vi "SFC_Get Model Label Template.vi"(8 "error in (no error)":errorcluster caption="错误输入（无错误）", 10 "Model":string, 11 "Traceability 引用句柄":refnum<k24>) -> (0 "error out":errorcluster caption="错误输出", 2 ".NET:System.Data.DataSet":T1={"CaseSensitive"=FALSE, "Container"=refnum, "DataSetName"="", "DefaultViewManager"=refnum, "DesignMode"=FALSE, "EnforceConstraints"=FALSE, "ExtendedProperties"=refnum, "HasErrors"=FALSE, "IsInitialized"=FALSE, "Locale"=refnum, "Namespace"="", "Prefix"="", "Relations"=refnum, "RemotingFormat"=0, "SchemaSerializationMode"=1, "Site"=refnum, "Tables"=refnum} {"SchemaSerializationMode" items=["IncludeSchema"=1, "ExcludeSchema"=2]; "RemotingFormat" items=["Xml", "Binary"]}, 3 "Traceability 引用句柄输出":refnum<k24>)   [LabVIEW 2014, in "Traceability.lvlib"]
uses:
  D:/webservice/Traceability.dll
  Traceability.dll
  System.Data
  Traceability.lvlib
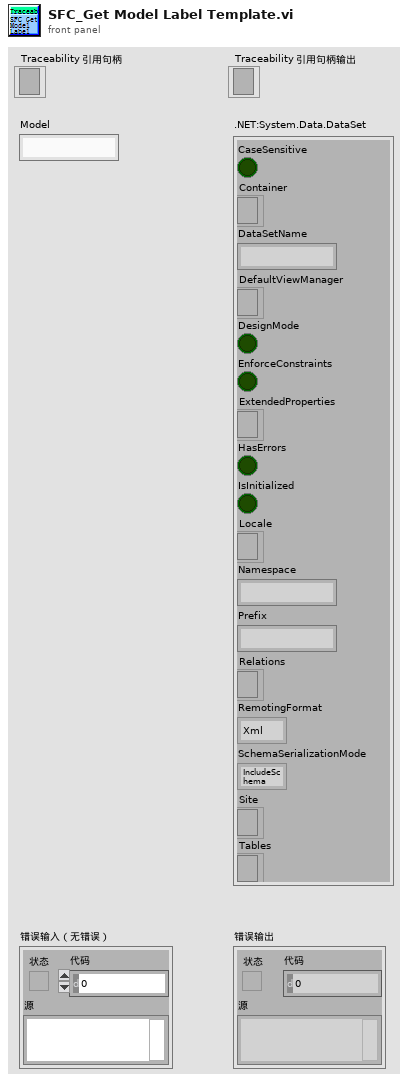
[diagram p1: front panel]
types:
  T1 = cluster{"CaseSensitive":bool, "Container":refnum<k24>, "DataSetName":string, "DefaultViewManager":refnum<k24>, "DesignMode":bool, "EnforceConstraints":bool, "ExtendedProperties":refnum<k24>, "HasErrors":bool, "IsInitialized":bool, "Locale":refnum<k24>, "Namespace":string, "Prefix":string, "Relations":refnum<k24>, "RemotingFormat":i32, "SchemaSerializationMode":i32, "Site":refnum<k24>, "Tables":refnum<k24>}
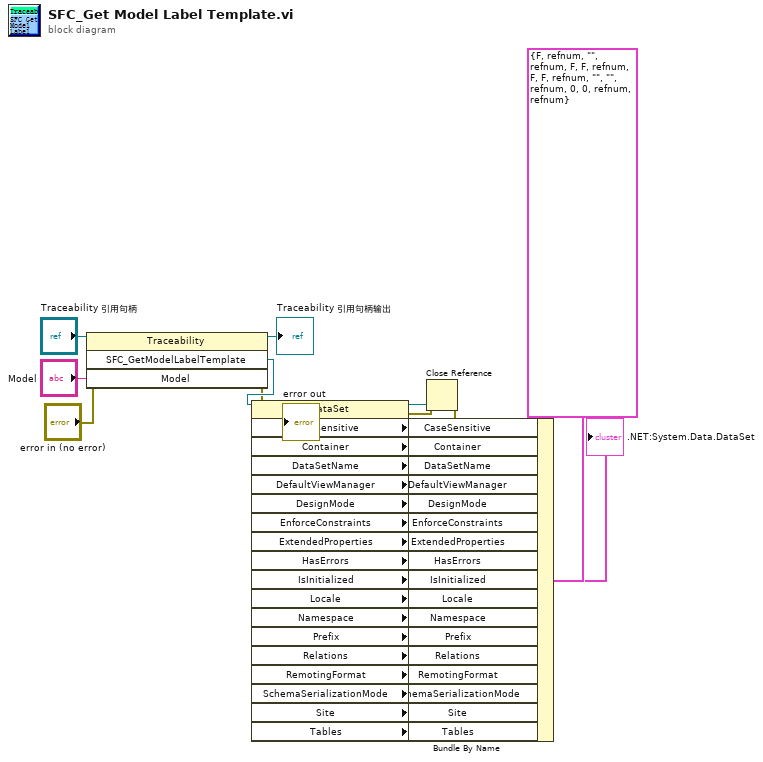
[diagram p0: block diagram]
diagram:
  n1 = invoke class="Traceability" method="SFC_GetModelLabelTemplate"(reference="Traceability 引用句柄", error in="error in (no error)", "Model"="Model") -> (reference out=→"Traceability 引用句柄输出":refnum<k24>, error out=w4:errorcluster, "SFC_GetModelLabelTemplate"=w25:refnum<k24>)  [unwired: 1 in, 1 out]
  n2 = property class="DataSet"(reference=w25, error in=w4) -> (reference out=w3:refnum<k24>, error out=w2:errorcluster, "CaseSensitive"=w22:bool, "Container"=w21:refnum<k24>, "DataSetName"=w20:string, "DefaultViewManager"=w19:refnum<k24>, "DesignMode"=w18:bool, "EnforceConstraints"=w17:bool, "ExtendedProperties"=w16:refnum<k24>, "HasErrors"=w15:bool, "IsInitialized"=w14:bool, "Locale"=w13:refnum<k24>, "Namespace"=w12:string, "Prefix"=w11:string, "Relations"=w10:refnum<k24>, "RemotingFormat"=w9:i32, "SchemaSerializationMode"=w8:i32, "Site"=w7:refnum<k24>, "Tables"=w6:refnum<k24>)
  n3 = Bundle By Name(cluster=T1 {"CaseSensitive"=FALSE, "Container"=refnum, "DataSetName"="", "DefaultViewManager"=refnum, "DesignMode"=FALSE, "EnforceConstraints"=FALSE, "ExtendedProperties"=refnum, "HasErrors"=FALSE, "IsInitialized"=FALSE, "Locale"=refnum, "Namespace"="", "Prefix"="", "Relations"=refnum, "RemotingFormat"=0, "SchemaSerializationMode"=0, "Site"=refnum, "Tables"=refnum} (".NET:System.Data.DataSet"), "CaseSensitive"=w22, "Container"=w21, "DataSetName"=w20, "DefaultViewManager"=w19, "DesignMode"=w18, "EnforceConstraints"=w17, "ExtendedProperties"=w16, "HasErrors"=w15, "IsInitialized"=w14, "Locale"=w13, "Namespace"=w12, "Prefix"=w11, "Relations"=w10, "RemotingFormat"=w9, "SchemaSerializationMode"=w8, "Site"=w7, "Tables"=w6) -> (→".NET:System.Data.DataSet":T1)
  n4 = Close Reference(reference=w3, error in (no error)=w2) -> (error out=→"error out":errorcluster)
